vi "Merge 8xI16 to 16xI16.vi"(0 "data in":i16[](array[numeric])=[0, 0, 0, 0, 0, 0, 0, 0], 2 "reset":bool, 5 "input valid":bool, 12 "ready for output (T)":bool=TRUE) -> (4 "data out":i16[](array[numeric]), 6 "output valid":bool, 14 "ready for input":bool)   [LabVIEW 2018, in "Streaming FPGA.lvlib"]
doc: "Merges two arrays of 8 I16s to an array of 16 I16s. Two data inputs generate a data output."
uses:
  Streaming FPGA.lvlib
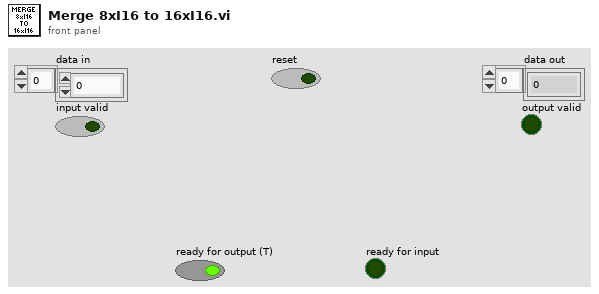
[diagram p1: front panel]
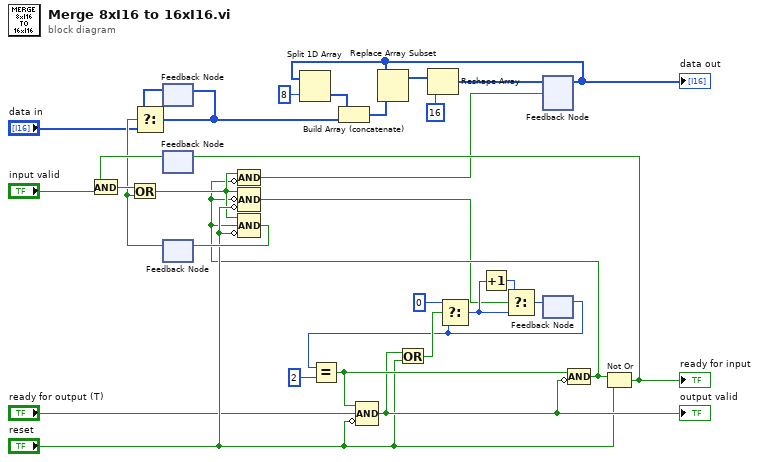
[diagram p0: block diagram]
diagram:
  n1 = feedback #1() -> (w27:i16[])  [unwired: 1 in]
  n2 = feedback #2() -> (w31:bool)  [unwired: 1 in]
  n3 = And(x=w31, y="input valid") -> (x .and. y?=w29:bool)
  n4 = feedback #3() -> (w28:bool)  [unwired: 1 in]
  n5 = Or(x=w29, y=w28) -> (x .or. y?=w4:bool)
  n6 = Select(t=w27, s=w28, f="data in") -> (s? t:f=w24:i16[])
  n7 = feedback-in #1(w24) -> ()
  n8 = feedback #4() -> (w10:i16[])  [unwired: 1 in]
  "data out" <- w10
  n9 = Split 1D Array(array=w10, index=8) -> (second subarray=w23:i16[])  [unwired: 1 out]
  n10 = Build Array (concatenate)(w23, w24) -> (w9:i16[])
  n11 = Replace Array Subset(array=w10, new element=w9) -> (w7:i16[])  [unwired: 1 in]
  n12 = Reshape Array(w7, 16 ("dimension size")) -> (w5:i16[])
  n13 = feedback #5() -> (w16:u16)  [unwired: 1 in]
  n14 = Equal?(x=w16, y=u16 2) -> (x = y?=w21:bool)
  n15 = Compound Arithmetic op=AND(w21, "ready for output (T)", invert "reset") -> (w14:bool)
  "output valid" <- w14
  n16 = Or(x=w14, y="reset") -> (x .or. y?=w17:bool)
  n17 = Select(t=u16 0, s=w17, f=w16) -> (s? t:f=w19:u16)
  n18 = Increment(x=w19) -> (x+1=w22:u16)
  n19 = Compound Arithmetic op=AND(w21, invert w14) -> (w3:bool)
  n20 = Compound Arithmetic op=AND(w4, invert w3) -> (w1:bool)
  n21 = Compound Arithmetic op=AND(w4, invert w3, invert "reset") -> (w2:bool)
  n22 = Compound Arithmetic op=AND(w4, w3, invert "reset") -> (w30:bool)
  n23 = feedback-in #3(w30) -> ()
  n24 = Select(t=w22, s=w2, f=w19) -> (s? t:f=w18:u16)
  n25 = feedback-in #4(w5, w1) -> ()
  n26 = feedback-in #5(w18) -> ()
  n27 = Not Or(1:"reset", 2:w3) -> (0:w15:bool)
  "ready for input" <- w15
  n28 = feedback-in #2(w15) -> ()
